vi "scaleFactor.vi"(11 "degrees":dbl) -> (3 "ticks":dbl)   [LabVIEW 2020]
uses:
  <vilib>/Analysis/coordinate.llb/Angle Range (Degree).ctl
  <vilib>/Analysis/coordinate.llb/Angle Units.ctl
  <vilib>/Analysis/coordinate.llb/Wrap Angle (scalar).vi
  <vilib>/Analysis/NI_AAL_Angle.lvlib
panel:
  in  "scale factor":dbl=5.6916
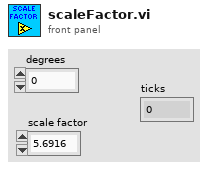
[diagram p1: front panel]
types:
  T1 = typedef "NI_AAL_Angle.lvlib/Angle Units.ctl" = i32
  T2 = typedef "NI_AAL_Angle.lvlib/Angle Range (Degree).ctl" = u16
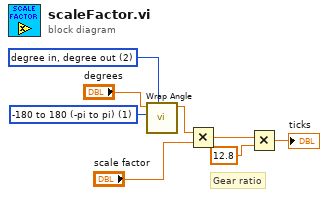
[diagram p0: block diagram]
diagram:
  w1 = T1 2 items=["radian in, radian out", "radian in, degree out", "degree in, degree out", "degree in, radian out"] ("angle units")
  w4 = T2 1 items=["none", "-180 to 180 (-pi to pi)", "0 to 360 (0 to 2pi)"] ("angle range")
  # "Gear ratio"
  n1 = call-poly <vilib>:"Wrap Angle.vi"("angle units"=w1, "angle range"=w4, "angle in"="degrees") -> ("angle out"=w3:dbl)  [unwired: 7 in, 1 out]
  n2 = Multiply(x=w3, y="scale factor") -> (x*y=w7:dbl)
  n3 = Multiply(x=w7, y=12.8) -> (x*y=→"ticks":dbl)
